vi "PH_Sixpack.PC RefSearch.vi"(0 "i ref in":refnum<vi>, 2 "axis":i32, 5 "error in (no error)":errorcluster) -> (14 "i ref out":refnum<vi>, 19 "error out":errorcluster)   [LabVIEW 2014, in "PH_Sixpack.lvlib"]
doc: "Sets ionformation to won attributes."
uses:
  PH_Sixpack.lvlib
  PH_Basics/PH_Common/PH_Common.lvlib
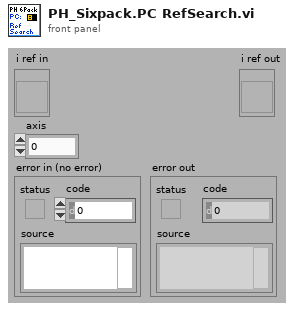
[diagram p1: front panel]
types:
  T1 = typedef "PH_Sixpack.lvlib/PH_Sixpack.i attribute.ctl" = cluster{"Information":cluster{"SixPack ID(0)":u16, "BaudRate(19200)":u16, "COM Port":enum32{"COM1", "COM2", "COM3", "COM4", "COM5", "COM6", "COM7", "COM8", "COM9"}, "HANDLE":i32}, "Serial Number":dbl, "Firmwareversion":dbl, "Axes":T2[], "Status":T14, "Axis to do a RefSearch":i32, "GUI Refs":cluster{"Information":refnum<vi>, "Serial Number":refnum<vi>, "Firmwareversion":refnum<vi>, "Status":refnum<vi>, "Axis to do a RefSearch":refnum<vi>, "Axes Configuration (Sixpack)":refnum<vi>, "Inputs":refnum<vi>, "PeriodicInterval [ms]":refnum<vi>}, "Constructor finished":bool, "Ignore Error":bool}
  T2 = typedef "PH_Sixpack.lvlib/PH_Sixpack.Axis Cluster.ctl" = cluster{"Config":T3, "To set?":cluster{"VmaxAmax":bool, "I max":bool, "VStartVminDivi":bool, "Ref Search Parameter":bool, "Stopswitch Limits":bool, "Axis Parameter":bool, "I Control":bool}}
  T3 = typedef "PH_Sixpack.lvlib/PH_Sixpack.Axis Configuration.ctl" = cluster{"VmaxAmax":T4, "I max (50%)":T5, "VStartVminDivi":T6, "Ref Search Parameter":T7, "Stopswitch Limits":T8, "Axis Parameter":T9, "I Control":T12}
  T4 = typedef "Sixpack - Driver.lvlib/VmaxAmax.ctl" = cluster{"VMax(511)":u16, "AMax(128)":u16}
  T5 = typedef "Sixpack - Driver.lvlib/PeakCurrent.ctl" = dbl
  T6 = typedef "Sixpack - Driver.lvlib/VStartVmin.ctl" = cluster{"VStart(5)":u16, "Vmin(4)":u16, "Div i (2)":enum8{"0", "1", "2", "3"}}
  T7 = typedef "Sixpack - Driver.lvlib/Ref Search Parameter.ctl" = cluster{"VRefMax(100)":u16, "DebouncingTime (22ms)":u8}
  T8 = typedef "Sixpack - Driver.lvlib/Stopswitch Limits.ctl" = cluster{"MinLeft(0)":u16, "MaxRight(1023)":u16}
  T9 = typedef "Sixpack - Driver.lvlib/Motor Parameter.ctl" = cluster{"Poslimit (6400)":u32, "P5 Bits":T10, "P6 Bits":T11}
  T10 = typedef "Sixpack - Driver.lvlib/MotorParameter_P5.ctl" = cluster{"MT_PI":bool, "MT_ROTARY":bool, "MT_AUTONULLCMD":bool, "MT_TESTNULL":bool, "MT_NULLLEFT":bool, "MT_NULLCENTRE":bool, "MT_STOPNULL":bool, "MT_FILTERSWITCH":bool}
  T11 = typedef "Sixpack - Driver.lvlib/MotorParameter_P6.ctl" = cluster{"MT_OPTIMIZEWAY":bool, "MT_FASTREF":bool, "MT_MECHREF":bool, "MT_DELAYTESTNULL":bool, "MT_STOPSOFT":bool, "MT_STOPNOREF":bool, "MT_NULLPOSITIVE":bool, "MUT_STOPFULSTEPS":bool}
  T12 = typedef "Sixpack - Driver.lvlib/Current Control.ctl" = cluster{"PowerDownDelay (500)":u16, "PowerDown (0%)":T13, "Standing (50%)":T13, "Running (75%)":T13, "Accelerating (100%)":T13}
  T13 = typedef "Sixpack - Driver.lvlib/Current.ctl" = enum8{"100%", "75%", "50%", "38%", "25%", "19%", "13%", "9%", "0%"}
  T14 = typedef "PH_Sixpack.lvlib/PH_Sixpack.Status.ctl" = enum32{"None", "Init", "Configure", "configured", "Close", "closed"}
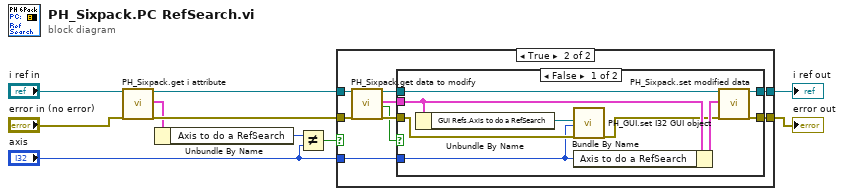
[diagram p0: block diagram]
diagram:
  n1 = call "PH_Sixpack.get i attribute.vi"("i ref in"="i ref in", "error in (no error)"="error in (no error)") -> ("i ref out"=w5:refnum<vi>, "i attribute"=w4:T1, "error out"=w7:errorcluster)  [unwired: 15 in]
  n2 = Unbundle By Name(w4) -> ("Axis to do a RefSearch"=w3:i32)
  n3 = Not Equal?(x=w3, y="axis") -> (x != y?=w1:bool)
  n4 = case shown="True" w1 {
    tunnel: [w12 w20] -> w10
    tunnel: [w11 w18] -> w8
    tunnel: w7 -> [w11 w15]
    tunnel: w5 -> [w12 w14]
    tunnel: "axis" -> [_ w13]
    frame False {
    }
    frame True {
      n5 = call "PH_Sixpack.get data to modify.vi"("i ref in"=w14, "error in (no error)"=w15) -> ("i ref out"=w21:refnum<vi>, "i attribute"=w17:T1, "timed out"=w16:bool, "error out"=w19:errorcluster)  [unwired: 14 in]
      n6 = case shown="False" w16 {
        tunnel: [w29 w32] -> w20
        tunnel: w21 -> [w28 w32]
        tunnel: [w30 w31] -> w18
        tunnel: w19 -> [w27 w31]
        tunnel: w17 -> [w25 _]
        tunnel: w13 -> [w22 _]
        frame False {
          n7 = Unbundle By Name(w25) -> ("GUI Refs.Axis to do a RefSearch"=w23:refnum<vi>)
          n8 = call "PH_GUI.set I32 GUI object.vi"("I32 GUI Ref"=w23, "value"=w22, "error in (no error)"=w27) -> ("error out"=w24:errorcluster)  [unwired: 16 in]
          n9 = Bundle By Name(cluster=w25, "Axis to do a RefSearch"=w22) -> (w26:T1)
          n10 = call "PH_Sixpack.set modified data.vi"("i ref in"=w28, "i attribute"=w26, "error in (no error)"=w24) -> ("i ref out"=w29:refnum<vi>, "error out"=w30:errorcluster)  [unwired: 15 in]
        }
        frame True {
        }
      }
    }
  }
  "error out" <- w8
  "i ref out" <- w10
